vi "PID Falcon test1.vi"(11 "refnum name":string="TEST Falcon 7") -> (2 "Stop 2":bool=TRUE, 10 "SP1:":dbl(slide)=31.0 min=0.0 max=0.0 scale=0.0..100.0)   [LabVIEW 2020]
doc: "This example demonstrates how to create a dual PID controller."
uses:
  <vilib>/Rock Robotics/WPI/ThirdParty/Phoenix-LabVIEW/Motor Controller/Controls/CTRE_Phoenix_MotorControl_ControlMode.ctl
  <vilib>/Rock Robotics/WPI/ThirdParty/Phoenix-LabVIEW/Motor Controller/Get/CTRE_Phoenix_MotorController_GetSelectedSensorData.vi
  <vilib>/addons/control/pid/pid.llb/PID (DBL).vi
  <vilib>/addons/control/pid/NI_PID_pid.lvlib
panel:
  out "x <= y?":bool
  out "SP error":dbl
  in  "error tol revs":dbl
  out "inches per rev":dbl
  in  "distance to travel":dbl(slide) scale=-24.0..24.0
  in  "encoder count/rev":dbl=2048.0 format="%#.3g"
  in  "wheel diameter (in)":dbl=1.0 format="%.3g"
  in  "Xmission gearing":dbl=1.0 format="%.3g"
  in  "derivative time (Td, min)":dbl=0.001 format="%.3f"
  in  "integral time (Ti, min)":dbl=0.1 format="%.3f"
  in  "proportional gain (Kc)":dbl=1.0 format="%.3f"
  out "MV1:":dbl(slide)=-0.5 scale=-100.0..100.0
  out "PV1:":dbl(slide)=1093.0 scale=0.0..100.0
  in  "Sampling Time dt (s)":dbl=0.05 min=0.001 step=0.01 format="%#.3p"
  in  "Stop":bool
  out "Process Variable and Setpoint":cluster{"Position (Raw Sensor Units)":i32, dbl}(graph)
  # "Overview: This example demonstrates how to create a dual PID controller.\nInstructions:\n1. Run the VI and observe the Process Variable (PV) following the Setpoint (SP) for both Controllers.\n2. Change the setpoint of one controller and verify that it does not affect the second controller.\n3. Click Stop to stop the VI."
  # "PID Parameters"
  # "Controller 1"
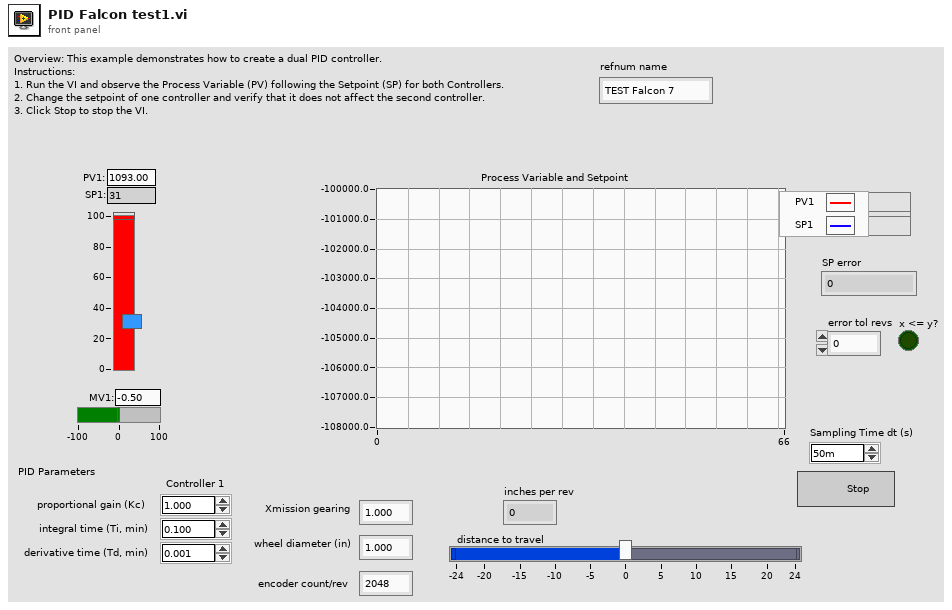
[diagram p1: front panel]
types:
  T1 = typedef "WPI_MotorControlDeviceRef.ctl" = cluster{"DeviceStatus":errorcluster, "Type":T2, "PWM":cluster{"PWM Channel":T3, "DeadBand":T4}, "CAN":cluster{"Device Number":u8, "SetOutput VI Ref":variant, "GetOutput VI Ref":variant, "Enable VI Ref":variant, "Disable VI Ref":variant, "Data":variant}, "Invert":bool, "DIO PWM":cluster{"PWM \"Enable\" Channel":T3, "DIOChannel":T5, "PWM Rate":dbl}}
  T2 = typedef "WPI_MotorControlType.ctl" = enum16{"PWM", "CAN", "DIO PWM"}
  T3 = typedef "FPGA_DIOPWMChannel.ctl" = enum8{"PWM 0", "PWM 1", "PWM 2", "PWM 3", "PWM 4", "PWM 5", "PWM 6", "PWM 7", "PWM 8", "PWM 9", "PWM MXP 0", "PWM MXP 1", "PWM MXP 2", "PWM MXP 3", "PWM MXP 4", "PWM MXP 5", "PWM MXP 6", "PWM MXP 7", "PWM MXP 8", "PWM MXP 9", "Invalid"}
  T4 = typedef "WPI_PWMDeadband.ctl" = cluster{"Name":string, "maxPositivePwm":i32, "minPositivePwm":i32, "centerPwm":i32, "maxNegativePwm":i32, "minNegativePwm":i32, "angularRange":u16}
  T5 = typedef "FPGA_DIOChannel.ctl" = enum8{"DIO 0", "DIO 1", "DIO 2", "DIO 3", "DIO 4", "DIO 5", "DIO 6", "DIO 7", "DIO 8", "DIO 9", "DIO MXP 0", "DIO MXP 1", "DIO MXP 2", "DIO MXP 3", "DIO MXP 4", "DIO MXP 5", "DIO MXP 6", "DIO MXP 7", "DIO MXP 8", "DIO MXP 9", "DIO MXP 10", "DIO MXP 11", "DIO MXP 12", "DIO MXP 13", "DIO MXP 14", "DIO MXP 15", "SPI Port CS1", "SPI Port CS2", "SPI Port CS3", "SPI Port MISO", "SPI Port MOSI", "Invalid"}
  T6 = typedef "CTRE_Phoenix_MotorControl_ControlMode.ctl" = u16
  T7 = cluster{"proportional gain (Kc)":dbl, "integral time (Ti, min)":dbl, "derivative time (Td, min)":dbl}
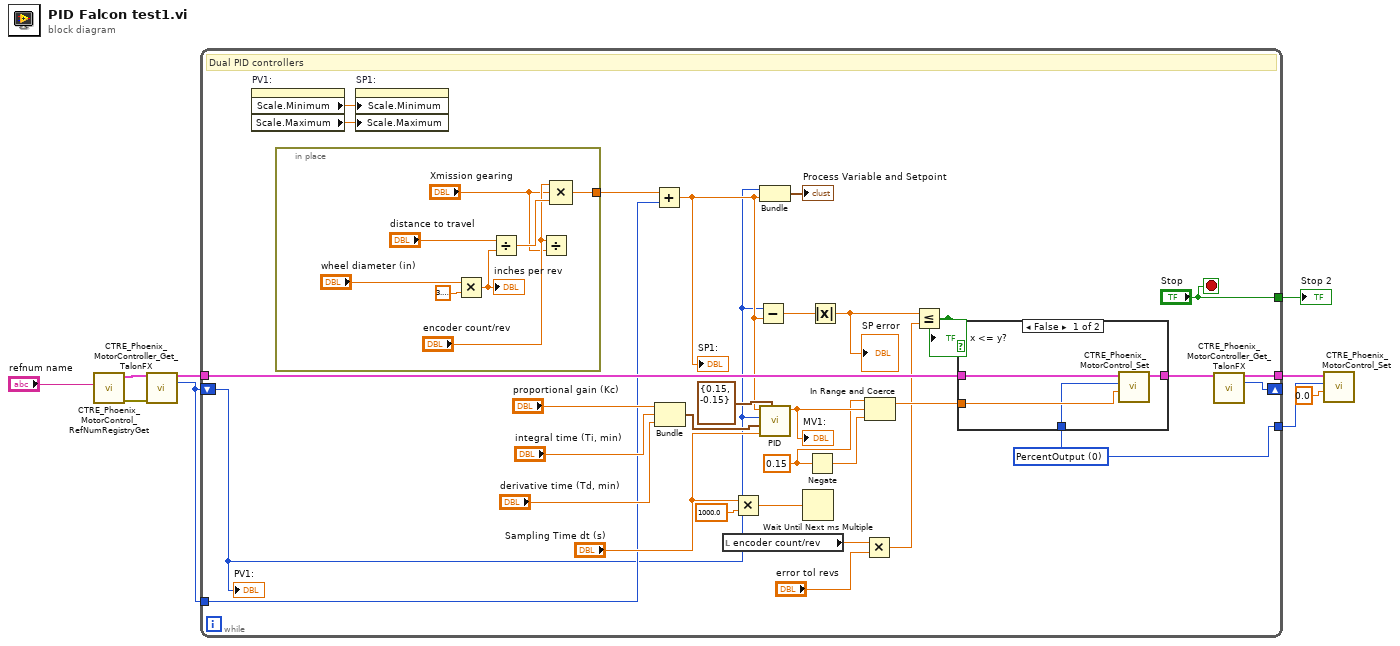
[diagram p0: block diagram]
diagram:
  n1 = call <vilib>:"CTRE_Phoenix_MotorControl_RefNumRegistryGet.vi"("refnum name"="refnum name") -> ("error out"=w2:errorcluster, "PhoenixMotorControlDevRef"=w8:T1)  [unwired: 9 in]
  n2 = call-poly <vilib>:"CTRE_Phoenix_MotorController_Get_TalonFX.vi"("PhoenixMotorControlDevRef"=w8, "error in"=w2) -> ("PhoenixMotorControlDevRef"=w9:T1, "Position (Raw Sensor Units)"=w1:i32)  [unwired: 10 in, 2 out]
  n3 = while {
    shift-left: w1 -> [w12]
    shift-right: [w22] -> _
    tunnel: w9 -> [w30]
    tunnel: ["Stop"] -> w6
    tunnel: [w23] -> w5
    tunnel: [w10] -> w4
    tunnel: w1 -> [w14]
    stop <- "Stop" stop-if-true
    w10 = T6 0 items=["PercentOutput"=0, "Position"=1, "Velocity"=2, "Current"=3, "Follower"=5, "MotionProfile"=6, "MotionMagic"=7, "MotionProfileArc"=10, "Disabled"=15] ("Control Mode")
    w25 = 0.15 ("upper limit")
    # "Dual PID controllers"
    n4 = property on="PV1:" class="Slide (strict)"() -> ("Scale.Minimum"=w39:dbl, "Scale.Maximum"=w38:dbl)  [unwired: 2 in, 2 out]
    n5 = in-place {
      in-place-border: [w48] -> w13
      n6 = Multiply(x="wheel diameter (in)", y=3.141592653589793) -> (x*y=w51:dbl)
      "inches per rev" <- w51
      n7 = Divide(x="distance to travel", y=w51) -> (x/y=w52:dbl)
      n8 = Divide(x="encoder count/rev", y="Xmission gearing") -> ()  [unwired: 1 out]
      n9 = Compound Arithmetic op=MULTIPLY("encoder count/rev", "Xmission gearing", w52) -> (w48:dbl)
    }
    n10 = property on="SP1:" class="Slide (strict)"("Scale.Minimum"=w39, "Scale.Maximum"=w38) -> ()  [unwired: 2 in, 2 out]
    n11 = Add(x=w13, y=w14) -> (x+y=w15:dbl)
    "SP1:" <- w15
    n12 = Bundle("proportional gain (Kc)"="proportional gain (Kc)", "integral time (Ti, min)"="integral time (Ti, min)", "derivative time (Td, min)"="derivative time (Td, min)") -> (w31:T7)  [unwired: 1 in]
    n13 = local read "encoder count/rev"() -> (w17:dbl)
    n14 = Multiply(x="Sampling Time dt (s)", y=1000.0) -> (x*y=w33:dbl)
    n15 = Subtract(x=w12, y=w15) -> (x-y=w21:dbl)
    n16 = Bundle("Position (Raw Sensor Units)"=w12, w15) -> (→"Process Variable and Setpoint":cluster{"Position (Raw Sensor Units)":i32, dbl})  [unwired: 1 in]
    n17 = call-poly <vilib>:"PID.vi"("output range"=cluster{"output high":dbl, "output low":dbl} {"output high"=0.15, "output low"=-0.15}, "dt (s)"="Sampling Time dt (s)", "PID gains"=w31, "process variable"=w12, "setpoint"=w15) -> ("output"=w28:dbl)  [unwired: 5 in, 1 out]
    "MV1:" <- w28
    n18 = Wait Until Next ms Multiple(millisecond multiple=w33) -> ()  [unwired: 1 out]
    n19 = Negate(x=w25) -> (-x=w24:dbl)
    n20 = Absolute Value(x=w21) -> (abs(x)=w20:dbl)
    "SP error" <- w20
    n21 = Multiply(x=w17, y="error tol revs") -> (x*y=w18:dbl)
    n22 = In Range and Coerce(upper limit=w25, x=w28, lower limit=w24) -> (coerced(x)=w26:dbl)  [unwired: 1 out]
    n23 = Less Or Equal?(x=w20, y=w18) -> (x <= y?=w11:bool)
    "x <= y?" <- w11
    n24 = case shown="False" w11 {
      tunnel: w30 -> [w44 w45]
      tunnel: [w43 w45] -> w29
      tunnel: w26 -> [w42 _]
      tunnel: w10 -> [w41 _]
      frame False {
        n25 = call <vilib>:"CTRE_Phoenix_MotorControl_Set.vi"("Output"=w42, "Control Mode"=w41, "PhoenixMotorControlDevRef"=w44) -> ("PhoenixMotorControlDevRef"=w43:T1)  [unwired: 7 in, 1 out]
      }
      frame True {
      }
    }
    n26 = call-poly <vilib>:"CTRE_Phoenix_MotorController_Get_TalonFX.vi"("PhoenixMotorControlDevRef"=w29) -> ("PhoenixMotorControlDevRef"=w23:T1, "Position (Raw Sensor Units)"=w22:i32)  [unwired: 11 in, 2 out]
    "PV1:" <- w12
  }
  "Stop 2" <- w6
  n27 = call <vilib>:"CTRE_Phoenix_MotorControl_Set.vi"("Output"=0.0, "Control Mode"=w4, "PhoenixMotorControlDevRef"=w5) -> ()  [unwired: 7 in, 2 out]
